vi "readFromXML.vi"(8 "error in (no error)":errorcluster, 10 "XMLin":string="<guideTargetConfiguration>  \n  <target>\n    <raDecParameters>\n      <declination>\n        <degreesDec>0</degreesDec>\n        <minutesArc>0</minutesArc>\n        <secondsArc>0</secondsArc>\n      </declination>\n      <equinoxPrefix>B</equinoxPrefix>\n      <equinoxYear>2000</equinoxYear>\n      <frame>FK4</frame>\n      <ra>\n        <hours>0</hours>\n        <minutes>0</minutes>\n        <seconds>0</seconds>\n      </ra>\n    </raDecParameters>\n    <parallax_Arcsec>0</parallax_Arcsec>\n    <properMotion>\n      <epochPM_Yr>2009</epochPM_Yr>\n      <pmdec_ArcsPYr>0</pmdec_ArcsPYr>\n      <pmra_SPYr>0</pmra_SPYr>\n    </properMotion>\n    <rv_kps>0</rv_kps>\n    <targetName/>\n    <difftrackRADec>\n      <dDec_ArcsPS>1</dDec_ArcsPS>\n      <dRA_sps>112.2</dRA_sps>\n    </difftrackRADec>\n  </target>\n  <targetConfigName>this is IT</targetConfigName>  \n  <wl_Microns>0.1</wl_Microns> \n  <commandID>1234</commandID>\n  <tcsErrorResponse>\n   <status>false</status>\n    <code>0</code>\n    <source/>\n  </tcsErrorResponse>\n</guideTargetConfiguration>", 11 "TargetConfiguration in":refnum<class "TargetConfiguration.lvclass">) -> (0 "error out":errorcluster, 3 "TargetConfiguration out":refnum<class "TargetConfiguration.lvclass">)   [LabVIEW 2022 SP3, in "TCSDataDefinitions.lvlib" / "TCSCommand.lvlib" / "TargetConfiguration.lvlib" / "TargetConfiguration.lvclass"]
uses:
  TargetConfiguration.lvclass
  <userlib>/Common/UnitsAndXML/FlattenItemWithUnitToXML/FlattenLengthToXML/LengthUnit.ctl
  TargetConfiguration.lvclass/TargetConfiguration.ctl
  TCSTcsCommand/TCSTcsCommand.lvclass
  Target/Target/Target.lvclass
  <userlib>/Common/UnitsAndXML/UnitsAndXML.lvlib
  <userlib>/Common/XML/XMLParser/XMLParser.lvclass
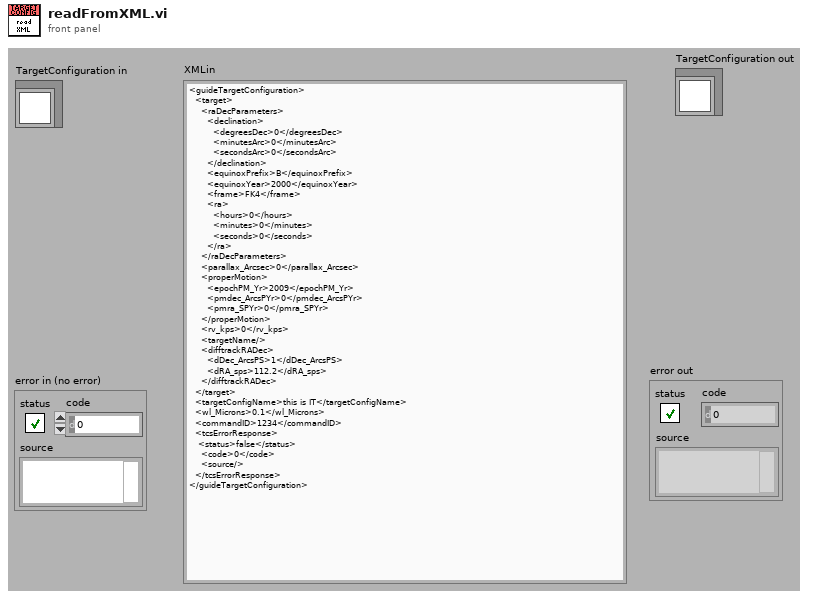
[diagram p1: front panel]
types:
  T1 = typedef "UnitsAndXML.lvlib/LengthUnit.ctl" = enum16{"m", "Angstrom", "AU", "chain", "cm", "cubit", "fathom", "fermi", "ft", "furlong", "hubble", "in", "ly", "mi", "mm", "rod", "um", "yd"}
  T2 = typedef "XML.lvlib/AttributeElements.ctl" = cluster{"attributeType":string, "attributeValue":string}
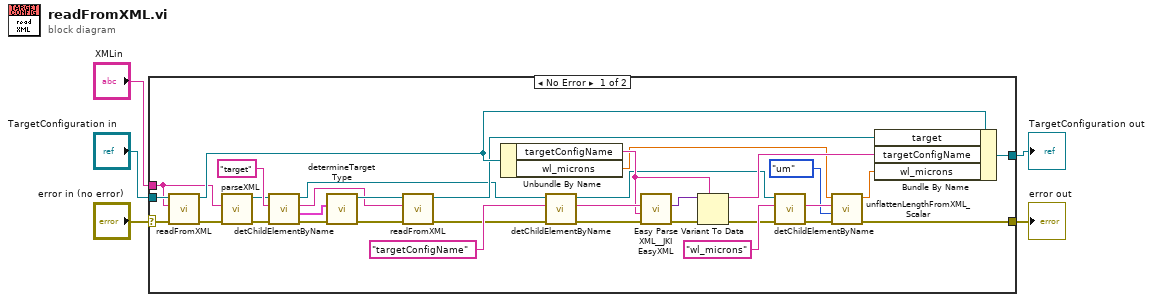
[diagram p0: block diagram]
diagram:
  n1 = case shown="No Error" "error in (no error)" {
    selector: "error in (no error)" -> [w37 w39]
    tunnel: [w31 w40] -> w2
    tunnel: "TargetConfiguration in" -> [w38 w40]
    tunnel: "XMLin" -> [w35 _]
    tunnel: [w17 w39] -> w1
    frame No Error {
      n2 = call-parent "readFromXML.vi"("error in (no error)"=w37, "XMLin"=w35, "TCSTcsCommand in"=w38) -> ("error out"=w34:errorcluster, "TCSTcsCommand out"=w36:refnum<class "TargetConfiguration.lvclass">)  [unwired: 7 in]
      n3 = call <userlib>:"parseXML.vi"("error in (no error)"=w34, "XMLString in"=w35) -> ("error out"=w15:errorcluster, "Element out"=w10:refnum<class "XMLParser.lvclass">)  [unwired: 8 in]
      n4 = call <userlib>:"detChildElementByName.vi"("error in (no error)"=w15, "childName"="target" ("ChildName"), "Element in"=w10) -> ("error out"=w13:errorcluster, "childAttributes"=w7:T2[], "childXML"=w6:string, "Element out"=w9:refnum<class "XMLParser.lvclass">)  [unwired: 5 in]
      n5 = call "determineTargetType.vi"("error in (no error)"=w13, "childAttributes"=w7) -> ("error out"=w11:errorcluster, "Target.lvclass"=w12:refnum<class "Target.lvclass">)  [unwired: 8 in]
      n6 = call-dynamic "readFromXML.vi"("error in (no error)"=w11, "XML in"=w6, "Target in"=w12) -> ("error out"=w30:errorcluster, "Target out"=w16:refnum<class "Target.lvclass">)  [unwired: 7 in]
      n7 = Unbundle By Name(w36) -> ("targetConfigName"=w25:string, "wl_microns"=w22:dbl[unit])
      n8 = call <userlib>:"detChildElementByName.vi"("error in (no error)"=w30, "childName"="targetConfigName" ("ChildName"), "Element in"=w9) -> ("error out"=w28:errorcluster, "childXML"=w29:string, "Element out"=w8:refnum<class "XMLParser.lvclass">)  [unwired: 5 in, 1 out]
      n9 = call <vilib>:"Easy Parse XML__JKI EasyXML.vi"("error in (no error)"=w28, "LabVIEW Data (Type)"=w25, "XML String"=w29) -> ("error out"=w26:errorcluster, "LabVIEW Data"=w27:variant)  [unwired: 7 in]
      n10 = Variant To Data(error in=w26, type=w25, Variant=w27) -> (data=w24:string, error out=w18:errorcluster)
      n11 = call <userlib>:"detChildElementByName.vi"("error in (no error)"=w18, "childName"="wl_microns" ("ChildName"), "Element in"=w8) -> ("error out"=w19:errorcluster, "childXML"=w23:string)  [unwired: 5 in, 2 out]
      n12 = call <userlib>:"unflattenLengthFromXML_Scalar.vi"("error in (no error)"=w19, "lengthUnitInXML"=LengthUnit."um", "xmlString"=w23, "lengthForType"=w22) -> ("error out"=w17:errorcluster, "length"=w21:dbl[unit])  [unwired: 6 in]
      n13 = Bundle By Name(cluster=w36, "target"=w16, "targetConfigName"=w24, "wl_microns"=w21) -> (w31:refnum<class "TargetConfiguration.lvclass">)
    }
    frame Error {
    }
  }
  "error out" <- w1
  "TargetConfiguration out" <- w2
